vi "convertsens.vi"(1 "Lockin input":i32, 2 "Voltage(T) Current(F)":bool) -> (0 "Sensitivity":dbl)   [LabVIEW 2013]
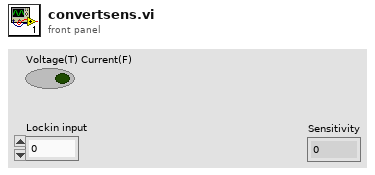
[diagram p1: front panel]
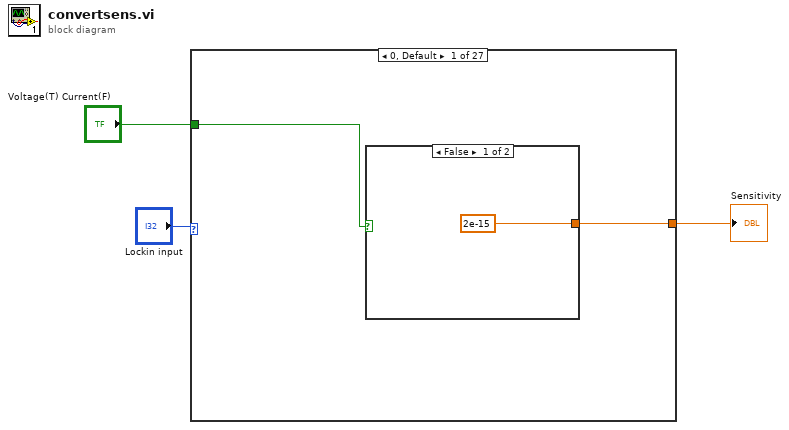
[diagram p0: block diagram]
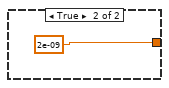
[diagram p2: hidden frame]
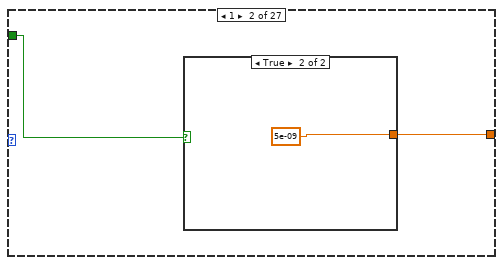
[diagram p3: hidden frame]
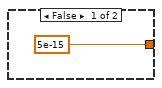
[diagram p4: hidden frame]
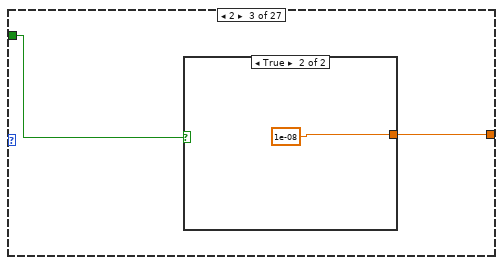
[diagram p5: hidden frame]
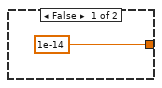
[diagram p6: hidden frame]
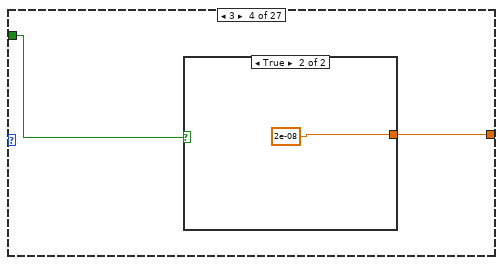
[diagram p7: hidden frame]
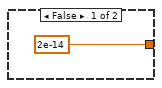
[diagram p8: hidden frame]
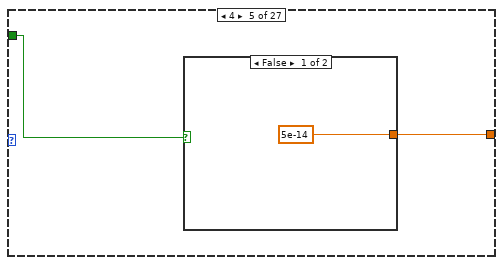
[diagram p9: hidden frame]
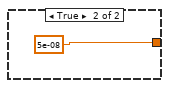
[diagram p10: hidden frame]
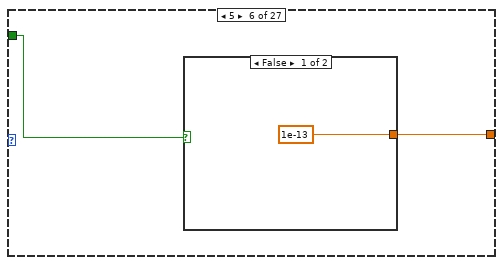
[diagram p11: hidden frame]
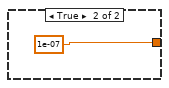
[diagram p12: hidden frame]
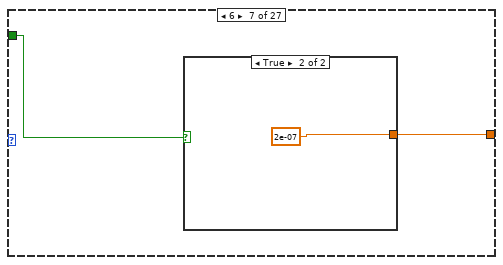
[diagram p13: hidden frame]
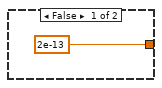
[diagram p14: hidden frame]
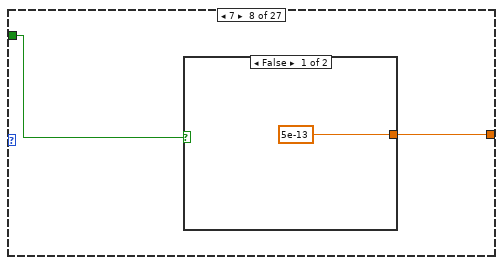
[diagram p15: hidden frame]
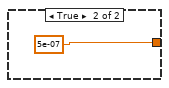
[diagram p16: hidden frame]
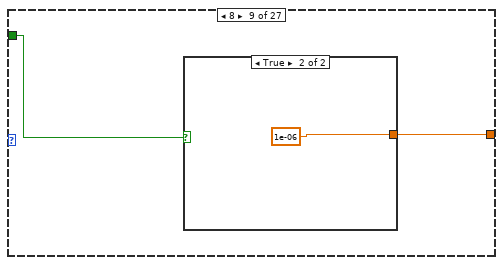
[diagram p17: hidden frame]
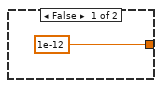
[diagram p18: hidden frame]
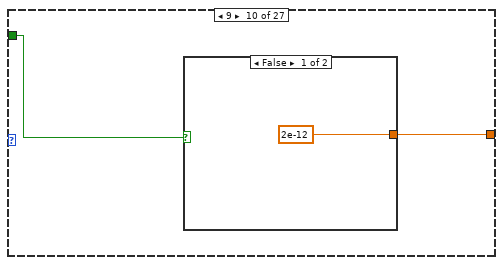
[diagram p19: hidden frame]
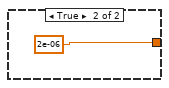
[diagram p20: hidden frame]
diagram:
  n1 = case shown="0, Default" "Lockin input" {
    tunnel: [w5 w9 w13 w17 w21 w25 w29 w33 w37 w41 w45 w49 w53 w57 w61 w65 w69 w73 w77 w81 w85 w89 w93 w97 w101 w105 w109] -> w2
    tunnel: "Voltage(T) Current(F)" -> [w4 w8 w12 w16 w20 w24 w28 w32 w36 w40 w44 w48 w52 w56 w60 w64 w68 w72 w76 w80 w84 w88 w92 w96 w100 w104 w108]
    frame 0, Default {
      n2 = case shown="False" w4 {
        tunnel: [2e-15 2e-09] -> w5
        frame False {
        }
        frame True {
        }
      }
    }
    frame 1 {
      n3 = case shown="True" w8 {
        tunnel: [5e-15 5e-09] -> w9
        frame False {
        }
        frame True {
        }
      }
    }
    frame 2 {
      n4 = case shown="True" w12 {
        tunnel: [1e-14 1e-08] -> w13
        frame False {
        }
        frame True {
        }
      }
    }
    frame 3 {
      n5 = case shown="True" w16 {
        tunnel: [2e-14 2e-08] -> w17
        frame False {
        }
        frame True {
        }
      }
    }
    frame 4 {
      n6 = case shown="False" w20 {
        tunnel: [5e-14 5e-08] -> w21
        frame False {
        }
        frame True {
        }
      }
    }
    frame 5 {
      n7 = case shown="False" w24 {
        tunnel: [1e-13 1e-07] -> w25
        frame False {
        }
        frame True {
        }
      }
    }
    frame 6 {
      n8 = case shown="True" w28 {
        tunnel: [2e-13 2e-07] -> w29
        frame False {
        }
        frame True {
        }
      }
    }
    frame 7 {
      n9 = case shown="False" w32 {
        tunnel: [5e-13 5e-07] -> w33
        frame False {
        }
        frame True {
        }
      }
    }
    frame 8 {
      n10 = case shown="True" w36 {
        tunnel: [1e-12 1e-06] -> w37
        frame False {
        }
        frame True {
        }
      }
    }
    frame 9 {
      n11 = case shown="False" w40 {
        tunnel: [2e-12 2e-06] -> w41
        frame False {
        }
        frame True {
        }
      }
    }
    frame 10 {
      n12 = case shown="True" w44 {
        tunnel: [5e-12 5e-06] -> w45
        frame False {
        }
        frame True {
        }
      }
    }
    frame 11 {
      n13 = case shown="False" w48 {
        tunnel: [1e-11 1e-05] -> w49
        frame False {
        }
        frame True {
        }
      }
    }
    frame 12 {
      n14 = case shown="True" w52 {
        tunnel: [2e-11 2e-05] -> w53
        frame False {
        }
        frame True {
        }
      }
    }
    frame 13 {
      n15 = case shown="False" w56 {
        tunnel: [5e-11 5e-05] -> w57
        frame False {
        }
        frame True {
        }
      }
    }
    frame 14 {
      n16 = case shown="True" w60 {
        tunnel: [1e-10 0.0001] -> w61
        frame False {
        }
        frame True {
        }
      }
    }
    frame 15 {
      n17 = case shown="False" w64 {
        tunnel: [2e-10 0.0002] -> w65
        frame False {
        }
        frame True {
        }
      }
    }
    frame 16 {
      n18 = case shown="True" w68 {
        tunnel: [5e-10 0.0005] -> w69
        frame False {
        }
        frame True {
        }
      }
    }
    frame 17 {
      n19 = case shown="False" w72 {
        tunnel: [1e-09 0.001] -> w73
        frame False {
        }
        frame True {
        }
      }
    }
    frame 18 {
      n20 = case shown="True" w76 {
        tunnel: [2e-09 0.002] -> w77
        frame False {
        }
        frame True {
        }
      }
    }
    frame 19 {
      n21 = case shown="False" w80 {
        tunnel: [5e-09 0.005] -> w81
        frame False {
        }
        frame True {
        }
      }
    }
    frame 20 {
      n22 = case shown="True" w84 {
        tunnel: [1e-08 0.01] -> w85
        frame False {
        }
        frame True {
        }
      }
    }
    frame 21 {
      n23 = case shown="False" w88 {
        tunnel: [2e-08 0.02] -> w89
        frame False {
        }
        frame True {
        }
      }
    }
    frame 22 {
      n24 = case shown="True" w92 {
        tunnel: [5e-08 0.05] -> w93
        frame False {
        }
        frame True {
        }
      }
    }
    frame 23 {
      n25 = case shown="False" w96 {
        tunnel: [1e-07 0.1] -> w97
        frame False {
        }
        frame True {
        }
      }
    }
    frame 24 {
      n26 = case shown="True" w100 {
        tunnel: [2e-07 0.2] -> w101
        frame False {
        }
        frame True {
        }
      }
    }
    frame 25 {
      n27 = case shown="False" w104 {
        tunnel: [5e-07 0.5] -> w105
        frame False {
        }
        frame True {
        }
      }
    }
    frame 26 {
      n28 = case shown="True" w108 {
        tunnel: [1e-06 1.0] -> w109
        frame False {
        }
        frame True {
        }
      }
    }
  }
  "Sensitivity" <- w2
